vi "OE1022_Query PLL&Overload.vi"(6 "Timeout":u32=1000, 8 "Error in (no error)":errorcluster caption="error out（no error）", 9 "Remote Mode":u16(ring) items=["USB"=0, "GPIB"=2], 11 "VISA resource name":refnum<visa-resource-name>) -> (0 "Error out":errorcluster caption="error out", 1 "Output String":string, 2 "OE1022_Query PLL&Overload":T1, 3 "VISA resource  out":refnum<visa-resource-name>)   [LabVIEW 2011]
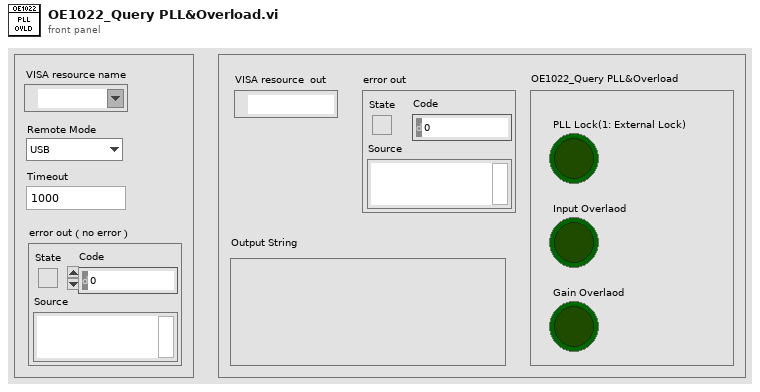
[diagram p1: front panel]
types:
  T1 = cluster{"PLL Lock(1: External Lock)":bool, "Input Overlaod":bool, "Gain Overlaod":bool}
  T2 = enum16{"ISRC", "IGND", "ICPL", "ILIN", "PHAS", "FMOD", "RSLP", "FREQ", "SWPT", "SLLM", "SULM", "SSLL", "SSLG", "STLM", "SWRM", "IRNG", "SENS", "RMOD", "OFLT", "OFSL", "SYNC", "DMOD", "HARM", "DARB", "SWVT", "SLVL", "SVLL", "SVUL", "SVSL", "SVSG", "SVTM", "SVRM", "RALL", "SNAP", "OUTP", "OAUX", "COUT", "CAUX", "COFP", "CEXP", "FPOP", "OEXP", "*IDN", "*RST", "OVLD", "INOV", "GNOV", "*PLL", "SSET", "RSET", "AGAN", "APHS", "ARSV", "ASCL", "EQCD", "EQCS", "SPED", "SRAT", "SLEN", "SSLE", "STRG", "SPRM", "STRD", "PAUS", "REST", "SPTS", "TRCA", "TEMP", "RSTU", "IHNZ", "DEQU", "SADD", "ARNG", "CSPE", "ISRCD", "IGNDD", "ICPLD", "ILIND", "PHASD", "FMODD", "RSLPD", "FREQD", "SWPTD", "SLLMD", "SULMD", "SSLLD", "SSLGD", "STLMD", "SWRMD", "SENSD", "RMODD", "OFLTD", "OFSLD", "SYNCD", "HARMD", "EQCDD", "EQCSD", "SNAPD", "OUTPD", "SWVTD", "SLVLD", "SVLLD", "SVULD", "SVSLD", "SVSGD", "SVTMD", "SVRMD", "SVDCD", "ARSVD", "AGAND", "APHSD", "ASCLD", "FPOPD", "CAUXD", "OEXPD", "SPEDD", "SRATD", "SLEND", "SSLED", "STRGD", "SPRMD", "STRDD", "PAUSD", "RESTD", "SPTSD", "TRCAD", "*IDND", "*RSTD", "INOVD", "GNOVD", "*PLLD", "SSETD", "RSETD"}
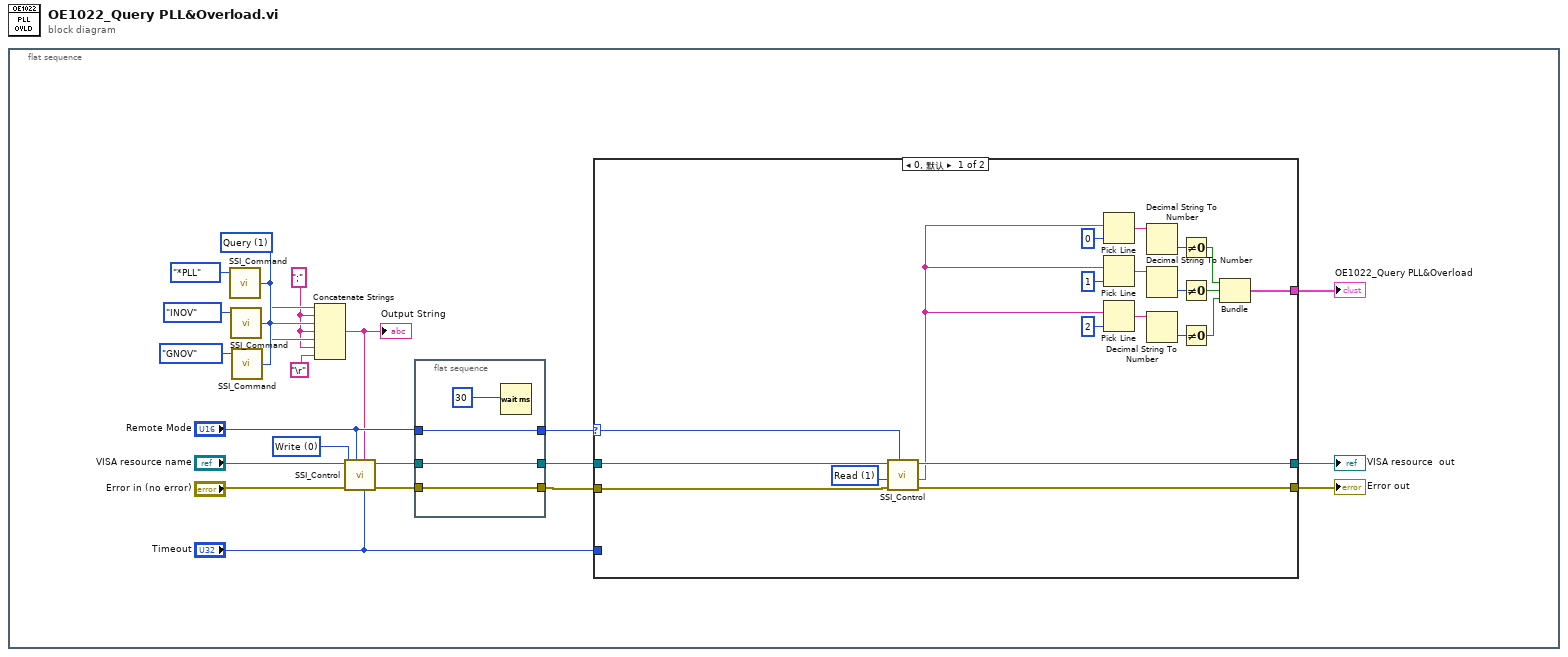
[diagram p0: block diagram]
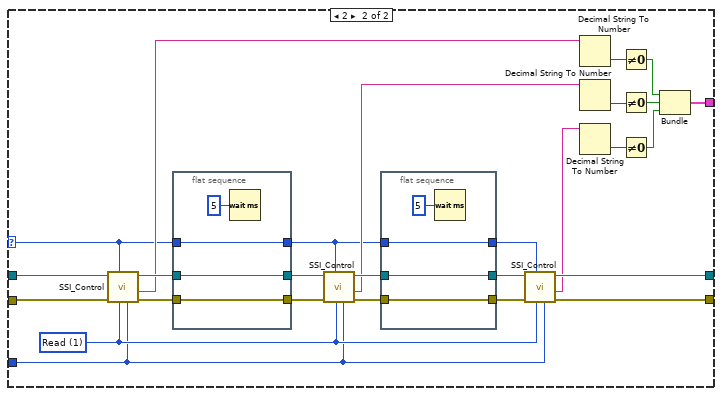
[diagram p2: hidden frame]
diagram:
  n1 = flat-sequence {
    frame #0 {
      w9 = ";"
      w13 = u16 1 items=["Set", "Query"] ("Opera")
      w22 = u16 0 items=["Write", "Read"] ("Control")
      n2 = call "SSI_Command.vi"("Opera"=w13, "Command Type"=T2."*PLL") -> ("Output string"=w12:string)  [unwired: 2 in]
      n3 = call "SSI_Command.vi"("Opera"=w13, "Command Type"=T2."INOV") -> ("Output string"=w11:string)  [unwired: 2 in]
      n4 = call "SSI_Command.vi"("Opera"=w13, "Command Type"=T2."GNOV") -> ("Output string"=w10:string)  [unwired: 2 in]
      n5 = Concatenate Strings(w12, w9, w11, w9, w10, w9, "\r") -> (w15:string)
      "Output String" <- w15
      n6 = call "SSI_Control.vi"("Tineout"="Timeout", "Write Buffer"=w15, "Remote Mode"="Remote Mode", "Error in (no error)"="Error in (no error)", "Control"=w22, "VISA resource name"="VISA resource name") -> ("Error out"=w19:errorcluster, "VISA resource  out"=w18:refnum<visa-resource-name>)  [unwired: 2 in, 2 out]
      n7 = flat-sequence {
        tunnel: [w82] -> w5
        tunnel: w19 -> [w82]
        tunnel: [w81] -> w6
        tunnel: w18 -> [w81]
        tunnel: "Remote Mode" -> [w80]
        tunnel: [w80] -> w7
        frame #0 {
          n8 = Wait (ms)(milliseconds to wait=30) -> ()  [unwired: 1 out]
        }
      }
      n9 = case shown="0, 默认" w7 {
        selector: w7 -> [w27 w49]
        tunnel: [w31 w67] -> w4
        tunnel: [w29 w58] -> w2
        tunnel: [w30 w57] -> w3
        tunnel: w6 -> [w25 w48]
        tunnel: w5 -> [w24 w47]
        tunnel: "Timeout" -> [_ w44]
        frame 0, Default {
          w28 = u16 1 items=["Write", "Read"] ("Control")
          n10 = call "SSI_Control.vi"("Remote Mode"=w27, "Error in (no error)"=w24, "Control"=w28, "VISA resource name"=w25) -> ("Error out"=w29:errorcluster, "Read Buffer"=w26:string, "VISA resource  out"=w30:refnum<visa-resource-name>)  [unwired: 4 in, 1 out]
          n11 = Pick Line(multi-line string=w26, line index=0 ("行索引")) -> (output string=w41:string)  [unwired: 1 in]
          n12 = Pick Line(multi-line string=w26, line index=1 ("行索引")) -> (output string=w42:string)  [unwired: 1 in]
          n13 = Pick Line(multi-line string=w26, line index=2 ("行索引")) -> (output string=w37:string)  [unwired: 1 in]
          n14 = Decimal String To Number(string=w41) -> (number=w32:i32)  [unwired: 2 in, 1 out]
          n15 = Decimal String To Number(string=w42) -> (number=w33:i32)  [unwired: 2 in, 1 out]
          n16 = Decimal String To Number(string=w37) -> (number=w34:i32)  [unwired: 2 in, 1 out]
          n17 = Not Equal To 0?(x=w32) -> (x != 0?=w40:bool)
          n18 = Not Equal To 0?(x=w33) -> (x != 0?=w43:bool)
          n19 = Not Equal To 0?(x=w34) -> (x != 0?=w35:bool)
          n20 = Bundle(w40, w43, w35) -> (w31:cluster{bool, bool, bool})  [unwired: 1 in]
        }
        frame 2 {
          w56 = u16 1 items=["Write", "Read"] ("Control")
          n21 = call "SSI_Control.vi"("Tineout"=w44, "Remote Mode"=w49, "Error in (no error)"=w47, "Control"=w56, "VISA resource name"=w48) -> ("Error out"=w66:errorcluster, "Read Buffer"=w53:string, "VISA resource  out"=w65:refnum<visa-resource-name>)  [unwired: 3 in, 1 out]
          n22 = flat-sequence {
            tunnel: [w78] -> w64
            tunnel: w66 -> [w78]
            tunnel: [w77] -> w63
            tunnel: w65 -> [w77]
            tunnel: w49 -> [w75]
            tunnel: [w75] -> w46
            frame #0 {
              n23 = Wait (ms)(milliseconds to wait=u32 5 ("等待时间（毫秒）")) -> ()  [unwired: 1 out]
            }
          }
          n24 = call "SSI_Control.vi"("Tineout"=w44, "Remote Mode"=w46, "Error in (no error)"=w64, "Control"=w56, "VISA resource name"=w63) -> ("Error out"=w61:errorcluster, "Read Buffer"=w52:string, "VISA resource  out"=w62:refnum<visa-resource-name>)  [unwired: 3 in, 1 out]
          n25 = flat-sequence {
            tunnel: [w74] -> w60
            tunnel: w61 -> [w74]
            tunnel: [w73] -> w59
            tunnel: w62 -> [w73]
            tunnel: w46 -> [w71]
            tunnel: [w71] -> w45
            frame #0 {
              n26 = Wait (ms)(milliseconds to wait=u32 5 ("等待时间（毫秒）")) -> ()  [unwired: 1 out]
            }
          }
          n27 = call "SSI_Control.vi"("Tineout"=w44, "Remote Mode"=w45, "Error in (no error)"=w60, "Control"=w56, "VISA resource name"=w59) -> ("Error out"=w58:errorcluster, "Read Buffer"=w55:string, "VISA resource  out"=w57:refnum<visa-resource-name>)  [unwired: 3 in, 1 out]
          n28 = Decimal String To Number(string=w53) -> (number=w50:i32)  [unwired: 2 in, 1 out]
          n29 = Decimal String To Number(string=w52) -> (number=w51:i32)  [unwired: 2 in, 1 out]
          n30 = Decimal String To Number(string=w55) -> (number=w54:i32)  [unwired: 2 in, 1 out]
          n31 = Not Equal To 0?(x=w50) -> (x != 0?=w69:bool)
          n32 = Not Equal To 0?(x=w51) -> (x != 0?=w70:bool)
          n33 = Not Equal To 0?(x=w54) -> (x != 0?=w68:bool)
          n34 = Bundle(w69, w70, w68) -> (w67:cluster{bool, bool, bool})  [unwired: 1 in]
        }
      }
      "Error out" <- w2
      "VISA resource  out" <- w3
      "OE1022_Query PLL&Overload" <- w4
    }
  }
